vi "publish.vi"(0 "HGF_SVService":refnum<class "HGF_SVService.lvclass">, 1 "typeDescriptor":string, 2 "data":variant, 3 "timeout in ms (-1)":i32, 5 "error in (no error)":errorcluster) -> (14 "dup HGF_SVService":refnum<class "HGF_SVService.lvclass">, 16 "rawData":variant, 17 "timed out?":bool, 19 "error out":errorcluster)   [LabVIEW 2012, in "HGF_SV.lvlib" / "HGF_SVService.lvclass"]
uses:
  HGF_SVService.lvclass
  HGF_BaseClasses/HGF_PVPublisher/HGF_PVPublisher.lvclass
  HGF_SVService.lvclass/HGF_SVService.ctl
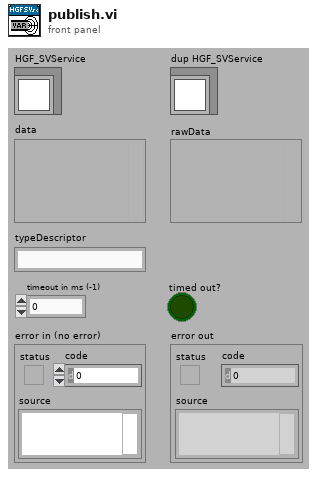
[diagram p1: front panel]
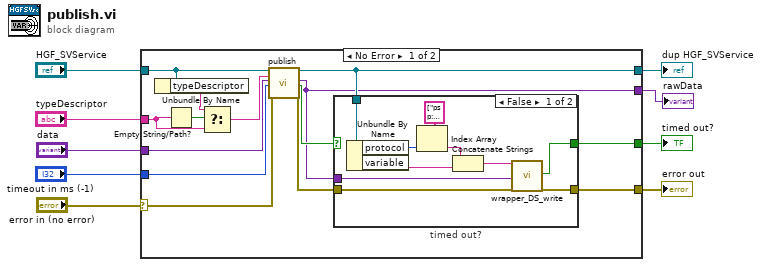
[diagram p0: block diagram]
diagram:
  n1 = case shown="No Error" "error in (no error)" {
    selector: "error in (no error)" -> [w22 w36]
    tunnel: [w20 w37] -> w9
    tunnel: [w18 w36] -> w8
    tunnel: "HGF_SVService" -> [w23 w37]
    tunnel: "data" -> [w21 _]
    tunnel: [w16 _] -> w4
    tunnel: [w15 _] -> w3
    tunnel: "typeDescriptor" -> [w13 _]
    tunnel: "timeout in ms (-1)" -> [w10 _]
    frame No Error {
      n2 = Unbundle By Name(w23) -> ("typeDescriptor"=w12:string)
      n3 = Empty String/Path?(string/path=w13) -> (empty?=w14:bool)
      n4 = Select(t=w12, s=w14, f=w13) -> (s? t:f=w11:string)
      n5 = call-parent "publish.vi"("HGF_PVPublisher"=w23, "typeDescriptor"=w11, "data"=w21, "timeout in ms (-1)"=w10, "error in (no error)"=w22) -> ("dup HGF_PVPublisher"=w20:refnum<class "HGF_SVService.lvclass">, "rawData"=w15:variant, "timed out?"=w17:bool, "error out"=w19:errorcluster)  [unwired: 11 out]
      n6 = case "timed out?" shown="False" w17 {
        selector: w17 -> [_ w35]
        tunnel: w20 -> [w33 _]
        tunnel: w15 -> [w27 _]
        tunnel: w19 -> [w26 w34]
        tunnel: [w25 w34] -> w18
        tunnel: [w24 w35] -> w16
        frame False {
          n7 = Unbundle By Name(w33) -> ("protocol"=w31:enum8{"psp", "opc"}, "variable"=w29:string)
          n8 = Index Array(array=string[] ["psp:", "opc:"], index=w31) -> (element=w30:string)
          n9 = Concatenate Strings(w30, w29) -> (w28:string)
          n10 = call "wrapper_DS_write.vi"("Connection In"=w28, "rawData"=w27, "error in"=w26) -> ("timed out"=w24:bool, "error out"=w25:errorcluster)  [unwired: 1 in, 14 out]
        }
        frame True {
        }
      }
    }
    frame Error {
    }
  }
  "error out" <- w8
  "dup HGF_SVService" <- w9
  "rawData" <- w3
  "timed out?" <- w4
